vi "Int Complex From Items.vi"(10 "Level Items":T1[](array[typedef])) -> (2 "Int Complex":cluster{"Number":i32[]}[](array[cluster]))   [LabVIEW 2019]
uses:
  Ancestor Class/Front Panel Container/Tree/Tree/Type Def/Tree Item.ctl
  Int 1D From Items.vi
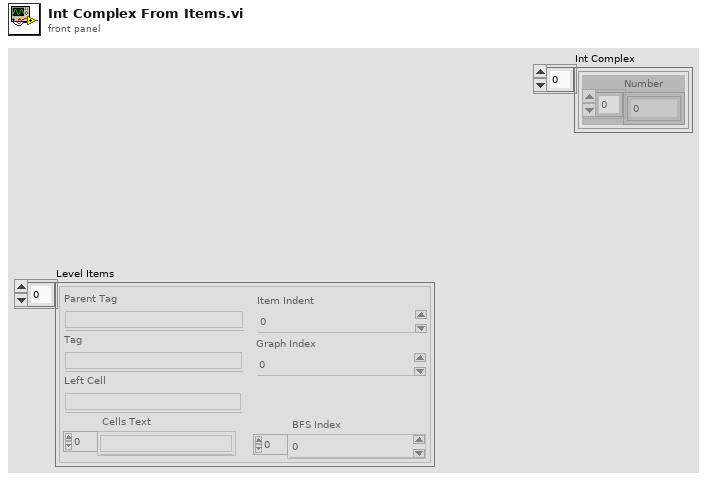
[diagram p1: front panel]
types:
  T1 = typedef "Tree Item.ctl" = cluster{"Parent Tag":string, "Tag":string, "Left Cell":string, "Cells Text":string[], "BFS Index":i32[], "Graph Index":i32, "Item Indent":i32}
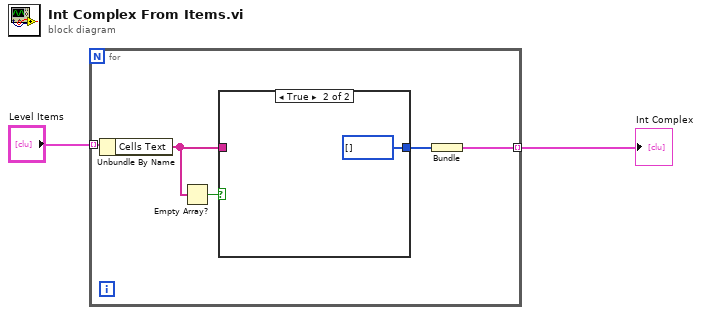
[diagram p0: block diagram]
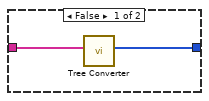
[diagram p2: hidden frame]
diagram:
  n1 = for {
    tunnel: "Level Items" -> [w7] mode=indexing
    tunnel: [w5] -> w1 mode=indexing
    n2 = Unbundle By Name(w7) -> ("Cells Text"=w4:string[])
    n3 = Empty Array?(array=w4) -> (empty?=w3:bool)
    n4 = case shown="True" w3 {
      tunnel: w4 -> [w9 _]
      tunnel: [w8 i32[] [] ("Number")] -> w6
      frame False {
        n5 = call-poly "Tree Converter.vi"("Child Text"=w9) -> ("Number"=w8:i32[])  [unwired: 10 in]
      }
      frame True {
      }
    }
    n6 = Bundle("Number"=w6) -> (w5:cluster{"Number":i32[]})  [unwired: 1 in]
  }
  "Int Complex" <- w1
